vi "MoverUmbralManual_Javi.vi"() -> ()   [LabVIEW 2019]
uses:
  Viejos/Alfredo LABVIEW/Set-up verificador ASICs/Lib Agilent 81160A/Agilent 81150/Agilent 81150.lvlib
panel:
  out "REGISTROS POST RESET":u16[](array[numeric]) format="%04x"
  in  "Numeric":u16 format="%04x"
  in  "stop":bool
  out "error out":errorcluster
  out "Write OK 2":bool
  out "Write OK":bool
  out "Reg 101-100\nCON 3 CANALES HABILITADOS":u32 format="%x"
  out "HANDLE":u32
  out "Error (\"1\" Error)":bool
  out "Todos":T1(array[cluster])=[{"Device Index"=0, "FT_FLAGS_OPENED"=TRUE, "FT_FLAGS_HISPEED"=TRUE, "Type"=6, "VID"=1027, "PID"=24592, "LocID"=1131585, "Serial Number"="CTAV2022A", "Description"="MI CTA TEST A", "FT_Handle"=433820616}, {"Device Index"=1, "FT_FLAGS_OPENED"=TRUE, "FT_FLAGS_HISPEED"=TRUE, "Type"=6, "VID"=1027, "PID"=24592, "LocID"=1131586, "Serial Number"="CTAV2022B", "Description"="MI CTA TEST B", "FT_Handle"=433822896}]
  out "Array CTA":T1(array[cluster])=[{"Device Index"=0, "FT_FLAGS_OPENED"=TRUE, "FT_FLAGS_HISPEED"=TRUE, "Type"=6, "VID"=1027, "PID"=24592, "LocID"=1131585, "Serial Number"="CTAV2022A", "Description"="MI CTA TEST A", "FT_Handle"=433820616}]
  # "REG99"
  # "REG102"
  # "REG96"
  # "REG97"
  # "REG98"
  # "REG100"
  # "REG101"
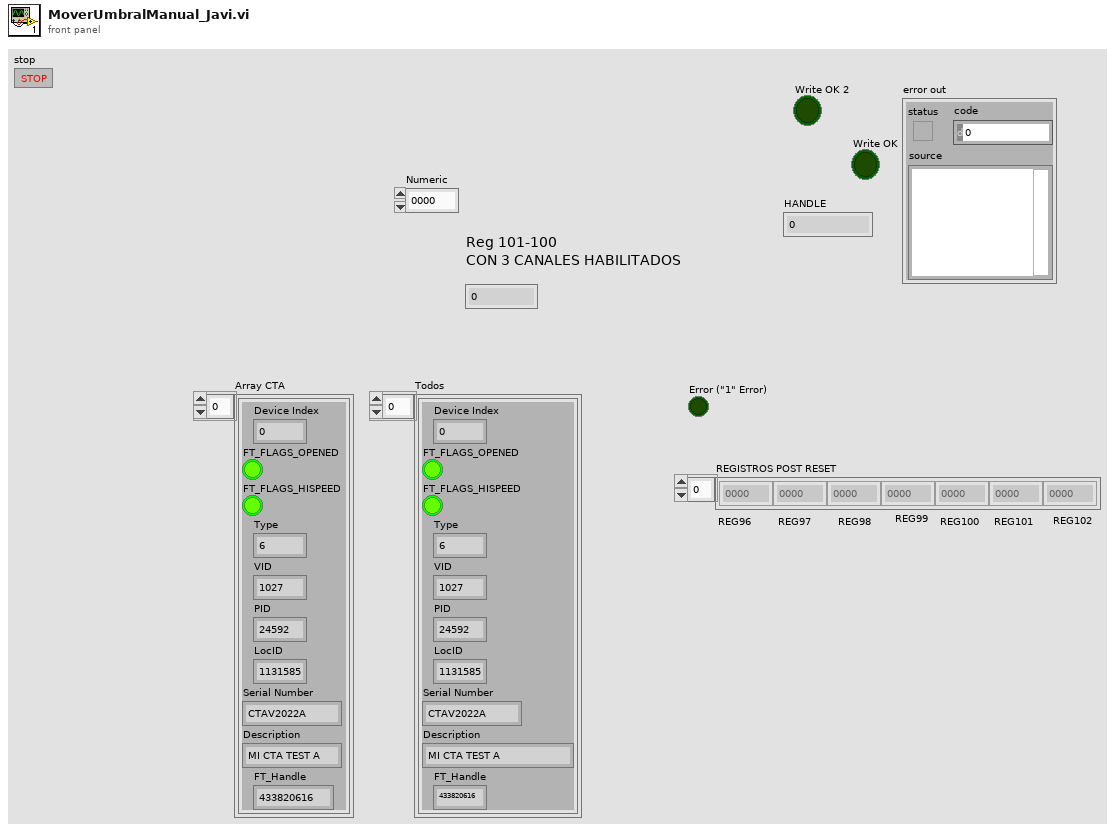
[diagram p1: front panel]
types:
  T1 = cluster{"Device Index":u32, "FT_FLAGS_OPENED":bool, "FT_FLAGS_HISPEED":bool, "Type":u32, "VID":u32, "PID":u32, "LocID":i32, "Serial Number":string, "Description":string, "FT_Handle":u32}[]
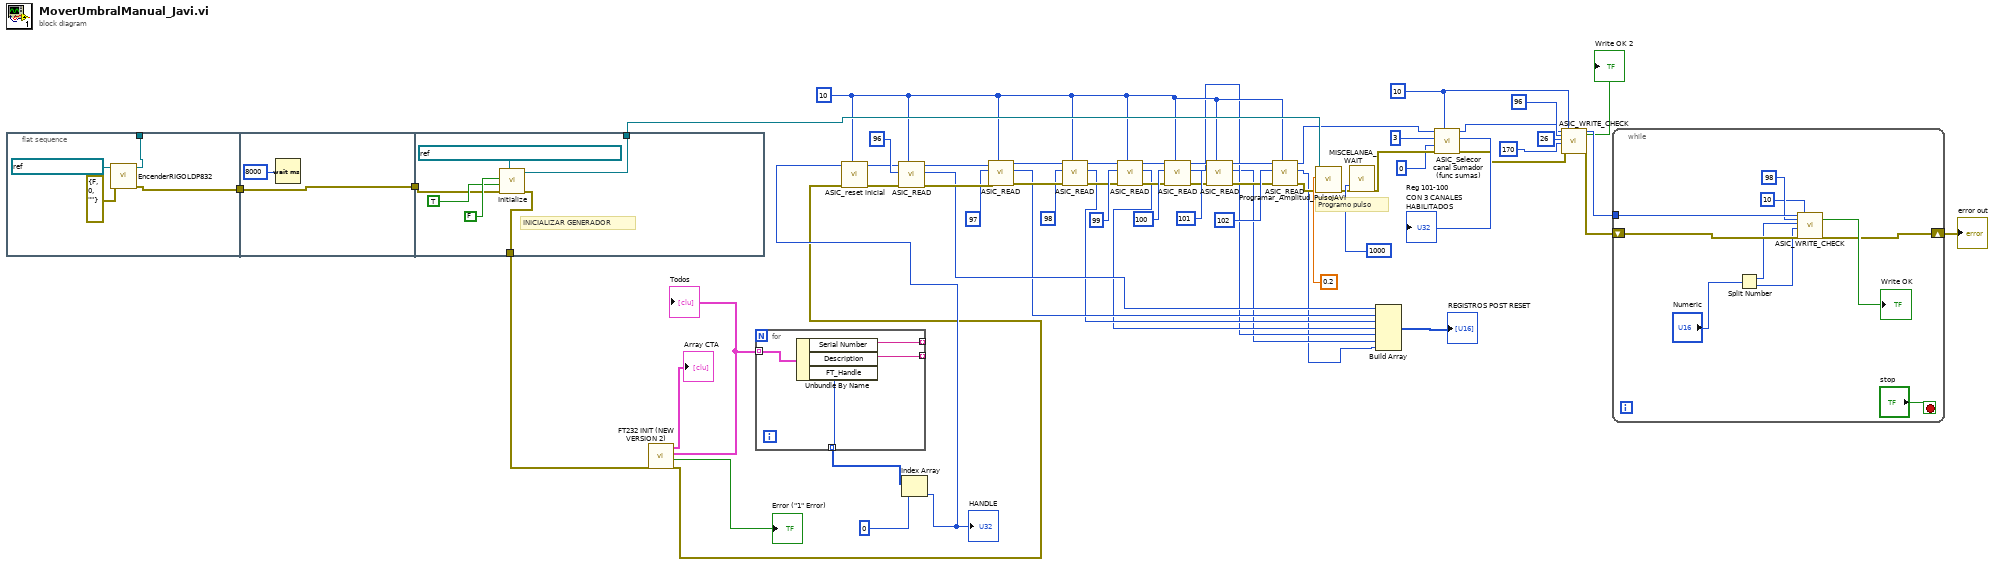
[diagram p0: block diagram]
diagram:
  w15 = u32 10 ("Espera acceso USB")
  w38 = u32 10 ("Espera acceso USB")
  # "Programo pulso"
  n1 = flat-sequence {
    tunnel: [w63] -> _
    tunnel: [w62] -> w60
    tunnel: w60 -> [w66]
    tunnel: [w66] -> w59
    tunnel: w59 -> [w70]
    tunnel: [w69] -> w53
    tunnel: [w67] -> w43
    frame #0 {
      n2 = call "EncenderRIGOLDP832.vi"("error in (no error)"=errorcluster {"status"=FALSE, "code"=0, "source"=""}, "VISA IN"=refnum<visa-resource-name> "FA_Rigol_DP832") -> ("error out"=w62:errorcluster, "VISA resource name out"=w63:refnum<visa-resource-name>)  [unwired: 8 in]
    }
    frame #1 {
      n3 = Wait (ms)(milliseconds to wait=u32 8000) -> ()  [unwired: 1 out]
    }
    frame #2 {
      # "INICIALIZAR GENERADOR"
      n4 = call "Initialize.vi"("error in (no error)"=w70, "Reset (True)"=TRUE, "ID Query (True)"=FALSE, "VISA resource name"=refnum<visa-resource-name> "USB0::0x0957::0x4108::MY51400682::INSTR") -> ("error out"=w69:errorcluster, "VISA resource name out"=w67:refnum<visa-resource-name>)  [unwired: 6 in]
    }
  }
  n5 = call "FT232 INIT (NEW VERSION 2).vi"("error in (no error)"=w53) -> ("error out"=w45:errorcluster, "Error (\"1\" Error)"=→"Error (\"1\" Error)":bool, "Todos"=w57:T1, "Array CTA"=→"Array CTA":T1)  [unwired: 7 in]
  "Todos" <- w57
  n6 = for {
    tunnel: w57 -> [w76] mode=indexing
    tunnel: [w75] -> _ mode=indexing
    tunnel: [w74] -> _ mode=indexing
    tunnel: [w73] -> w58 mode=indexing
    n7 = Unbundle By Name(w76) -> ("Serial Number"=w75:string, "Description"=w74:string, "FT_Handle"=w73:u32)
  }
  n8 = Index Array(array=w58, index=0) -> (element=w46:u32)
  "HANDLE" <- w46
  n9 = call "ASIC_reset inicial.vi"("Espera acceso USB"=w15, "error in"=w45, "ftHandle_in"=w46) -> ("error out"=w30:errorcluster, "ftHandle_out"=w31:u32)  [unwired: 7 in]
  n10 = call "ASIC_READ.vi"("Espera acceso USB"=w15, "error in"=w30, "Direccion Registro Asic"=u8 96, "ftHandle_in"=w31) -> ("error out"=w28:errorcluster, "Valor Asic"=w8:u16, "ftHandle_out"=w29:u32)  [unwired: 5 in]
  n11 = call "ASIC_READ.vi"("Espera acceso USB"=w15, "error in"=w28, "Direccion Registro Asic"=u8 97, "ftHandle_in"=w29) -> ("error out"=w26:errorcluster, "Valor Asic"=w7:u16, "ftHandle_out"=w20:u32)  [unwired: 5 in]
  n12 = call "ASIC_READ.vi"("Espera acceso USB"=w15, "error in"=w26, "Direccion Registro Asic"=u8 98, "ftHandle_in"=w20) -> ("error out"=w14:errorcluster, "Valor Asic"=w6:u16, "ftHandle_out"=w19:u32)  [unwired: 5 in]
  n13 = call "ASIC_READ.vi"("Espera acceso USB"=w15, "error in"=w14, "Direccion Registro Asic"=u8 99, "ftHandle_in"=w19) -> ("error out"=w13:errorcluster, "Valor Asic"=w5:u16, "ftHandle_out"=w18:u32)  [unwired: 5 in]
  n14 = call "ASIC_READ.vi"("Espera acceso USB"=w15, "error in"=w13, "Direccion Registro Asic"=u8 100, "ftHandle_in"=w18) -> ("error out"=w12:errorcluster, "Valor Asic"=w4:u16, "ftHandle_out"=w17:u32)  [unwired: 5 in]
  n15 = call "ASIC_READ.vi"("Espera acceso USB"=w15, "error in"=w12, "Direccion Registro Asic"=u8 101, "ftHandle_in"=w17) -> ("error out"=w11:errorcluster, "Valor Asic"=w3:u16, "ftHandle_out"=w16:u32)  [unwired: 5 in]
  n16 = call "ASIC_READ.vi"("Espera acceso USB"=w15, "error in"=w11, "Direccion Registro Asic"=u8 102, "ftHandle_in"=w16) -> ("error out"=w10:errorcluster, "Valor Asic"=w1:u16, "ftHandle_out"=w9:u32)  [unwired: 5 in]
  n17 = call "Programar_Amplitud_PulsoJAVI.vi"("error in (no error)"=w10, "Numeric"=0.2, "VISA Refnum in"=w43) -> ("Error OUT"=w51:errorcluster)  [unwired: 7 in, 1 out]
  n18 = call "MISCELANEA_WAIT.vi"("ms wait IN"=u32 1000, "Error IN"=w51) -> ("Error OUT"=w49:errorcluster)  [unwired: 16 in, 1 out]
  n19 = Build Array(w8, w7, w6, w5, w4, w3, w1) -> (→"REGISTROS POST RESET":u16[])
  n20 = call "ASIC_Selecor canal Sumador (func sumas).vi"("Espera acceso USB"=w38, "error in"=w49, "Sumador"=u8 0, "Modo"=u8 3, "ftHandle_in"=w9) -> ("error out"=w37:errorcluster, "Reg 101-100"=→"Reg 101-100\nCON 3 CANALES HABILITADOS":u32, "ftHandle_out"=w39:u32)  [unwired: 3 in, 1 out]
  n21 = call "ASIC_WRITE_CHECK.vi"("ftHandle_in"=w39, "Direccion Registro Asic"=u8 96, "Byte Alto"=u8 26, "Byte Bajo"=u8 170, "error in"=w37, "Espera acceso USB 2"=w38) -> ("ftHandle_out"=w36:u32, "Write OK"=→"Write OK 2":bool, "error out"=w34:errorcluster)  [unwired: 11 in]
  n22 = while {
    tunnel: w36 -> [w86]
    shift-right: [w81] -> w33
    shift-left: w34 -> [w85]
    stop <- "stop" stop-if-true
    n23 = Split Number(x="Numeric") -> (hi(x)=w78:u8, lo(x)=w77:u8)
    n24 = call "ASIC_WRITE_CHECK.vi"("ftHandle_in"=w86, "Direccion Registro Asic"=u8 98, "Byte Alto"=w78, "Byte Bajo"=w77, "error in"=w85, "Espera acceso USB 2"=u32 10) -> ("Write OK"=→"Write OK":bool, "error out"=w81:errorcluster)  [unwired: 11 in, 1 out]
  }
  "error out" <- w33
